vi "Check CRC-16.vi"(8 "error in (no error)":errorcluster caption="error in（no error）", 9 "CRC-16-H":u8 format="%.0x", 10 "CRC-16-L":u8 format="%.0x", 11 "Data In":u8[](array[numeric]) format="%.0x") -> (0 "error out":errorcluster, 3 "Check Result":bool)   [LabVIEW 2014, in "ALPHA5 RS485.lvlib"]
uses:
  ALPHA5 RS485.lvlib
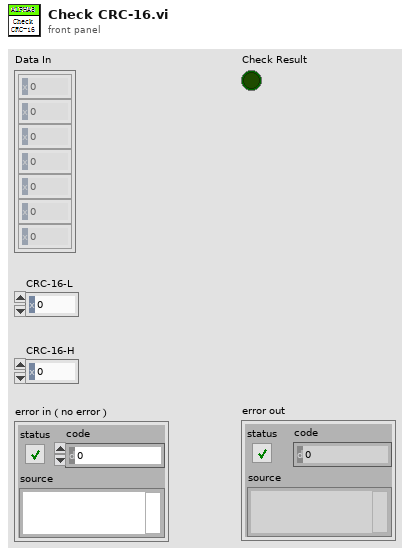
[diagram p1: front panel]
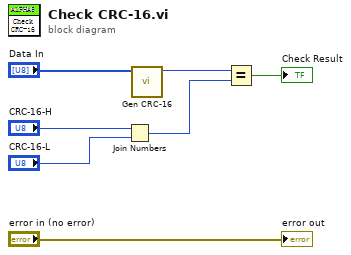
[diagram p0: block diagram]
diagram:
  n1 = Join Numbers(hi="CRC-16-H", lo="CRC-16-L") -> ((hi.lo)=w3:u16)
  n2 = call "Gen CRC-16.vi"("Data In"="Data In") -> ("CRC-16-Result"=w4:u16)  [unwired: 7 in, 3 out]
  n3 = Equal?(x=w4, y=w3) -> (x = y?=→"Check Result":bool)
  "error out" <- "error in (no error)"
